vi "ISweep_skeleton.vi"(1 "DMM1 GPIB address":string="11", 2 "DMM2 GPIB address":string="22", 3 "Main Temperature Controller GPIB address":string="15", 6 "Measurement wai time (ms)":dbl=150.0, 12 "Setpoint temperature (K)":dbl=50.0 format="%.3f", 14 "File Name":string="testing.txt", 15 "File Path":path=path "c:/data", 16 "Voltage resolution (mV)":dbl=1.0 format="%.1f", 18 "Allowable temperature deviation (K)":dbl=0.005 format="%.4f", 19 "Number of voltage measurements\nbetween temperature check":dbl=10.0) -> ()   [LabVIEW 2014]
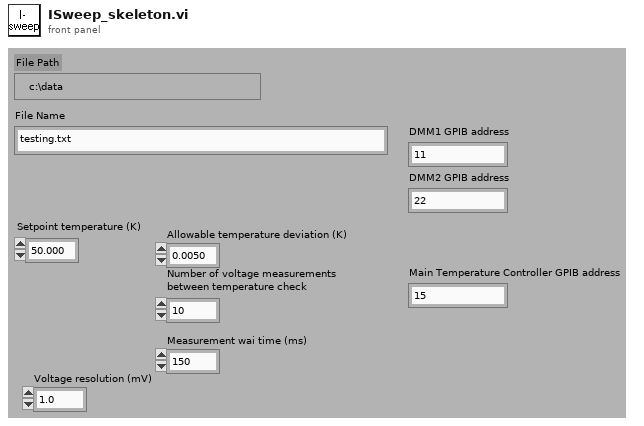
[diagram p1: front panel]
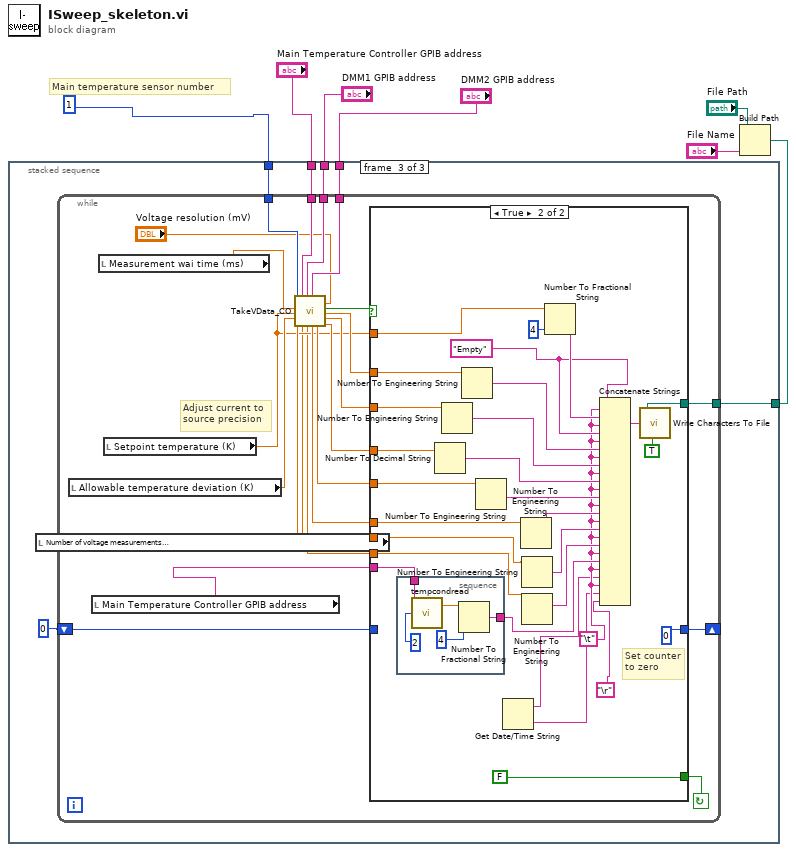
[diagram p0: block diagram]
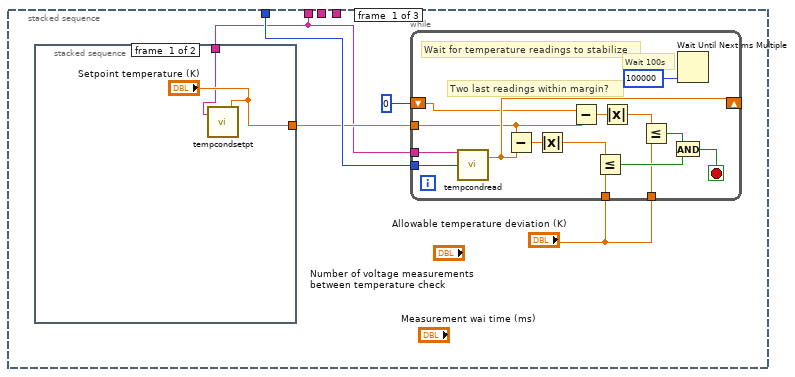
[diagram p2: hidden frame]
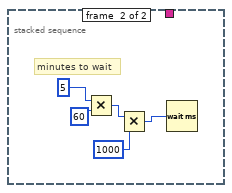
[diagram p3: hidden frame]
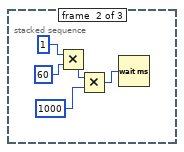
[diagram p4: hidden frame]
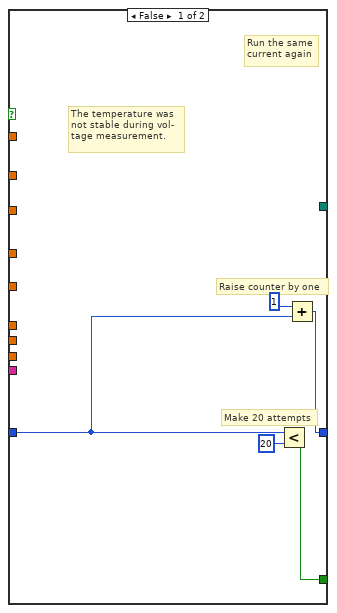
[diagram p5: hidden frame]
diagram:
  # "Main temperature sensor number"
  n1 = Build Path(base path="File Path", name or relative path="File Name") -> (appended path=w7:path)
  n2 = stacked-sequence {
    tunnel: w7 -> [_ _ w42]
    tunnel: "DMM1 GPIB address" -> [_ _ w45]
    tunnel: 1 -> [w11 _ w43]
    tunnel: "Main Temperature Controller GPIB address" -> [w9 _ w44]
    tunnel: "DMM2 GPIB address" -> [_ _ w40]
    frame #0 {
      n3 = stacked-sequence {
        tunnel: w9 -> [w28 _]
        tunnel: ["Setpoint temperature (K)" _] -> w10
        frame #0 {
          n4 = call "tempcondsetpt.vi"("Set Point"="Setpoint temperature (K)", "GPIB Address"=w28) -> ()  [unwired: 1 in, 1 out]
        }
        frame #1 {
          # "minutes to wait"
          n5 = Multiply(x=5, y=60) -> (x*y=w32:i32)
          n6 = Multiply(x=w32, y=1000) -> (x*y=w34:i32)
          n7 = Wait (ms)(milliseconds to wait=w34) -> ()  [unwired: 1 out]
        }
      }
      n8 = while {
        tunnel: w10 -> [w13]
        tunnel: "Allowable temperature deviation (K)" -> [w14]
        tunnel: "Allowable temperature deviation (K)" -> [w15]
        tunnel: w9 -> [w16]
        tunnel: w11 -> [w17]
        shift-left: 0 -> [w18]
        shift-right: [w19] -> _
        stop <- w24 stop-if-true
        # "Two last readings within margin?"
        # "Wait for temperature readings to stabilize"
        # "Wait 100s"
        n9 = call "tempcondread.vi"("Ring"=w17, "GPIB Address"=w16) -> ("Temperature"=w19:dbl)  [unwired: 1 in, 1 out]
        n10 = Subtract(x=w13, y=w19) -> (x-y=w26:dbl)
        n11 = Absolute Value(x=w26) -> (abs(x)=w23:dbl)
        n12 = Subtract(x=w18, y=w13) -> (x-y=w22:dbl)
        n13 = Less Or Equal?(x=w23, y=w15) -> (x <= y?=w25:bool)
        n14 = Absolute Value(x=w22) -> (abs(x)=w21:dbl)
        n15 = Less Or Equal?(x=w21, y=w14) -> (x <= y?=w20:bool)
        n16 = And(x=w20, y=w25) -> (x .and. y?=w24:bool)
        n17 = Wait Until Next ms Multiple(millisecond multiple=100000) -> ()  [unwired: 1 out]
      }
    }
    frame #1 {
      n18 = Multiply(x=1, y=60) -> (x*y=w36:i32)
      n19 = Multiply(x=w36, y=1000) -> (x*y=w38:i32)
      n20 = Wait (ms)(milliseconds to wait=w38) -> ()  [unwired: 1 out]
    }
    frame #2 {
      n21 = while {
        tunnel: w40 -> [w63]
        shift-left: 0 -> [w64]
        shift-right: [w65] -> _
        tunnel: w42 -> [w67]
        tunnel: w43 -> [w60]
        tunnel: w44 -> [w61]
        tunnel: w45 -> [w62]
        stop <- w66 continue-if-true
        # "Adjust current to\nsource precision"
        n22 = local read "Number of voltage measurements\nbetween temperature check"() -> (w52:dbl)
        n23 = local read "Allowable temperature deviation (K)"() -> (w53:dbl)
        n24 = local read "Main Temperature Controller GPIB address"() -> (w46:string)
        n25 = local read "Measurement wai time (ms)"() -> (w50:dbl)
        n26 = local read "Setpoint temperature (K)"() -> (w51:dbl)
        n27 = call "TakeVData_CO.vi"("Sensor"=w60, "Measurement wait time (ms)"=w50, "Setpoint temperature (K)"=w51, "Allowable deviation (K)"=w53, "Number of voltage measurements\nbetween temperature check"=w52, "Temperature Controller GPIB address"=w61, "DMM (to sample) GPIB address"=w62, "DMM2 GPIB address"=w63, "Cutoff (mV)"="Voltage resolution (mV)") -> ("Mean Temp (C)"=w49:dbl, "Temp error (C)"=w48:dbl, "Voltage error 2 (V)"=w55:dbl, "Mean Voltage 2 (V)"=w56:dbl, "Temperature stable?"=w59:bool, "Mean Voltage 1 (V)"=w54:dbl, "Voltage error 1 (V)"=w58:dbl, "Number of measurements"=w57:dbl)  [unwired: 3 in]
        n28 = case shown="True" w59 {
          tunnel: w67 -> [_ w100]
          tunnel: [w71 FALSE] -> w66
          tunnel: [w70 0] -> w65
          tunnel: w64 -> [w68 _]
          tunnel: w51 -> [_ w92]
          tunnel: w54 -> [_ w85]
          tunnel: w58 -> [_ w91]
          tunnel: w57 -> [_ w90]
          tunnel: w56 -> [_ w87]
          tunnel: w55 -> [_ w86]
          tunnel: w46 -> [_ w80]
          tunnel: w49 -> [_ w82]
          tunnel: w48 -> [_ w81]
          frame False {
            # "Raise counter by one"
            # "Run the same\ncurrent again"
            # "The temperature was\nnot stable during vol-\ntage measurement."
            # "Make 20 attempts"
            n29 = Less?(x=w68, y=20) -> (x < y?=w71:bool)
            n30 = Add(x=1, y=w68) -> (x+y=w70:i32)
          }
          frame True {
            w77 = "Empty"
            w76 = "\t"
            # "Set counter\nto zero"
            n31 = stacked-sequence {
              tunnel: w80 -> [w103]
              tunnel: [w102] -> w79
              frame #0 {
                n32 = call "tempcondread.vi"("Ring"=2, "GPIB Address"=w103) -> ("Temperature"=w106:dbl)  [unwired: 1 in, 1 out]
                n33 = Number To Fractional String(number=w106, precision (6)=4) -> (F-format string=w102:string)  [unwired: 2 in]
              }
            }
            n34 = Number To Decimal String(number=w90) -> (decimal integer string=w95:string)  [unwired: 1 in]
            n35 = Number To Engineering String(4:w91) -> (0:w98:string)  [unwired: 3 in]
            n36 = Number To Engineering String(4:w85) -> (0:w99:string)  [unwired: 3 in]
            n37 = Number To Engineering String(4:w87) -> (0:w89:string)  [unwired: 3 in]
            n38 = Get Date/Time String() -> (date string=w75:string, time string=w74:string)  [unwired: 3 in]
            n39 = Number To Engineering String(4:w86) -> (0:w88:string)  [unwired: 3 in]
            n40 = Number To Engineering String(4:w82) -> (0:w84:string)  [unwired: 3 in]
            n41 = Number To Engineering String(4:w81) -> (0:w83:string)  [unwired: 3 in]
            n42 = Number To Fractional String(number=w92, precision (6)=4) -> (F-format string=w93:string)  [unwired: 2 in]
            n43 = Concatenate Strings(w77, w76, w93, w76, w77, w76, w99, w76, w98, w76, w95, w76, w89, w76, w88, w76, w84, w76, w83, w76, w79, w76, w75, w76, w74, "\r") -> (w97:string)
            n44 = call <vilib>:"Write Characters To File.vi"("append to file? (new file:F)"=TRUE, "character string"=w97, "file path (dialog if empty)"=w100) -> ()  [unwired: 2 in, 1 out]
          }
        }
      }
    }
  }
